vi "valesForward.vi"(2 "threshold":dbl, 3 "iPeaksLocation":dbl[](array[numeric]), 4 "filteredSignal":dbl[](array[numeric]), 5 "iPeak":i32) -> (0 "ValesAmplitude":dbl, 1 "iValesLocation":dbl format="%.2f")   [LabVIEW 2011]
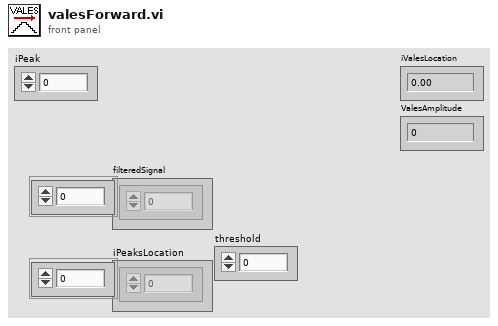
[diagram p1: front panel]
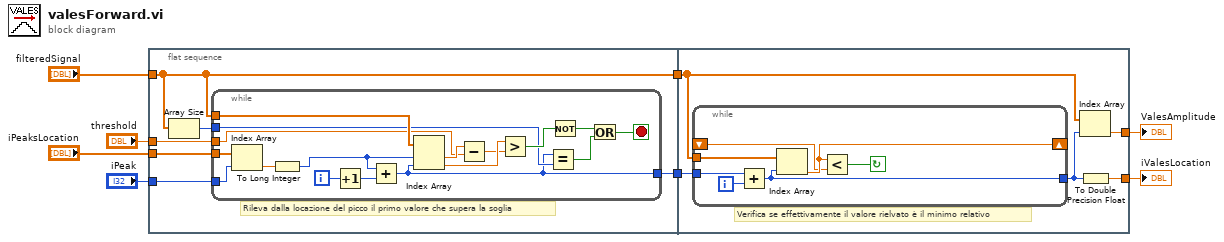
[diagram p0: block diagram]
diagram:
  n1 = flat-sequence {
    tunnel: "filteredSignal" -> [w10]
    tunnel: "iPeaksLocation" -> [w14]
    tunnel: "iPeak" -> [w9]
    tunnel: "threshold" -> [w13]
    tunnel: [w12] -> w4
    tunnel: [w10] -> w3
    tunnel: w4 -> [w36]
    tunnel: w3 -> [w35]
    tunnel: [w32] -> w2
    tunnel: [w33] -> w1
    frame #0 {
      # "Rileva dalla locazione del picco il primo valore che supera la soglia"
      n2 = Array Size(array=w10) -> (size(s)=w11:i32)
      n3 = while {
        tunnel: w10 -> [w29]
        tunnel: w14 -> [w31]
        tunnel: w9 -> [w30]
        tunnel: w13 -> [w23]
        tunnel: [w17] -> w12
        tunnel: w11 -> [w18]
        i -> [w28]
        stop <- w20 stop-if-true
        n4 = Index Array(array=w31, index=w30) -> (element=w27:dbl)
        n5 = To Long Integer(number=w27) -> (32bit integer=w25:i32)
        n6 = Increment(x=w28) -> (x+1=w26:i32)
        n7 = Add(x=w25, y=w26) -> (x+y=w17:i32)
        n8 = Index Array(array=w29, index #1=w25, index #2=w17) -> (element #1=w24:dbl, element #2=w22:dbl)
        n9 = Subtract(x=w24, y=w23) -> (x-y=w21:dbl)
        n10 = Greater?(x=w22, y=w21) -> (0:w19:bool)
        n11 = Equal?(x=w17, y=w18) -> (x = y?=w16:bool)
        n12 = Not(x=w19) -> (.not. x?=w15:bool)
        n13 = Or(x=w15, y=w16) -> (x .or. y?=w20:bool)
      }
    }
    frame #1 {
      # "Verifica se effettivamente il valore rielvato è il minimo relativo"
      n14 = while {
        tunnel: w36 -> [w42]
        tunnel: w35 -> [w43]
        shift-right: [w40] -> _
        shift-left: _ -> [w39]
        tunnel: [w37] -> w34
        i -> [w41]
        stop <- w38 continue-if-true
        n15 = Add(x=w42, y=w41) -> (x+y=w37:i32)
        n16 = Index Array(array=w43, index=w37) -> (element=w40:dbl)
        n17 = Less?(x=w40, y=w39) -> (x < y?=w38:bool)
      }
      n18 = Index Array(array=w35, index=w34) -> (element=w33:dbl)
      n19 = To Double Precision Float(number=w34) -> (double precision float=w32:dbl)
    }
  }
  "iValesLocation" <- w2
  "ValesAmplitude" <- w1
